vi "Update Tree.vi"(7 "Tree":refnum<vi>, 8 "error in (no error)":errorcluster, 11 "GenericGuiAI in":refnum<class "GenericGuiAI.lvclass">) -> (0 "error out":errorcluster, 3 "GenericGuiAI out":refnum<class "GenericGuiAI.lvclass">)   [LabVIEW 2020, in "VolatusDAQGenericGUI.lvlib" / "GenericGuiAI.lvclass"]
uses:
  GenericGuiAI.lvclass
  AI Tree Entry.ctl
  Channel Entry.ctl
  GenericGuiAI.lvclass/GenericGuiAI.ctl
  lv-vecto/Vecto/GroupAbstract/GroupAbstract.lvclass/GroupAbstract.ctl
  lv-vecto/Vecto/Channel/Channel.lvclass/Channel.ctl
  lv-vecto/Vecto/Group/Group.lvclass
  C:/dev/lv20CE/relink/lv-vecto/Vecto/GroupAbstract/GroupAbstract.lvclass
  lv-vecto/Vecto/GroupAbstract/Channel Info by Index.vi
  lv-vecto/Vecto/GroupAbstract/GroupAbstract.lvclass
  lv-vecto/Vecto/Group Config/Group Config.lvclass
  lv-vecto/Vecto/Channel/Channel.lvclass
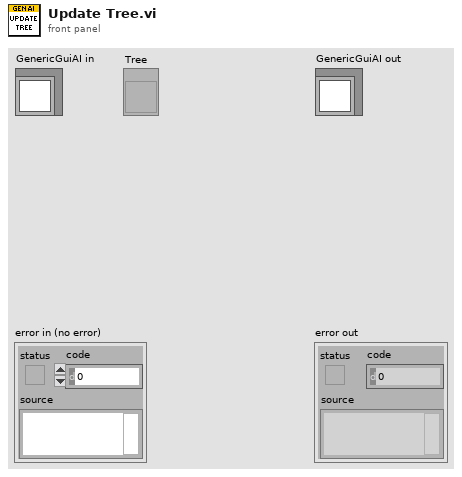
[diagram p1: front panel]
types:
  T1 = typedef "VolatusDAQGenericGUI.lvlib/GenericGuiAI.lvclass/AI Tree Entry.ctl" = cluster{"Hierarchy":string[], "Name":string, "Is Channel":bool, "Channel":T2}
  T2 = typedef "VolatusDAQGenericGUI.lvlib/GenericGuiAI.lvclass/Channel Entry.ctl" = cluster{"Resource":string, "Value":dbl, "Timestamp":dbl, "Raw":dbl}
  T3 = typedef "VectoConfig.lvlib/Group Info.ctl" = cluster{"System":string, "Cluster":string, "Node":string, "Task":string, "Name":string}
  T4 = typedef "VectoConfig.lvlib/Channel Info.ctl" = cluster{"Name":string, "Group":string, "Owning Node":string, "Owning Task":string, "Resource":string}
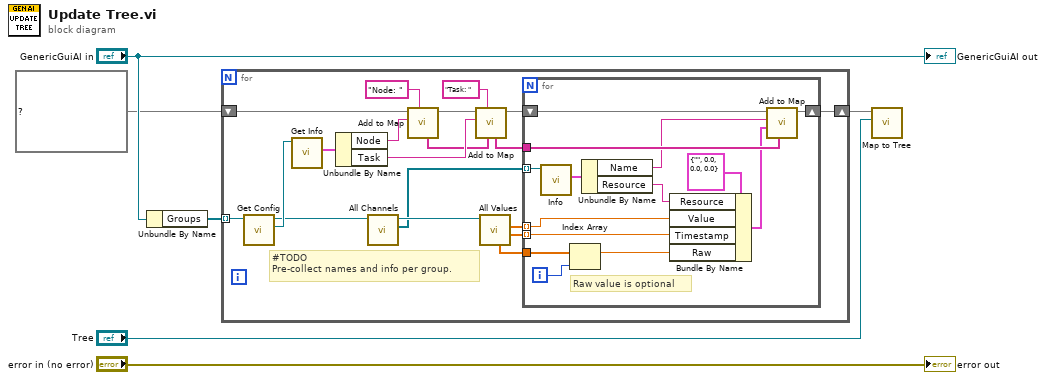
[diagram p0: block diagram]
diagram:
  n1 = Unbundle By Name("GenericGuiAI in") -> ("Groups"=w3:refnum<class "Group.lvclass">[])
  n2 = for {
    shift-right: [w10] -> w2
    shift-left: map{string[], T1} {} ("Map in") -> [w25]
    tunnel: w3 -> [w24] mode=indexing
    # "#TODO\nPre-collect names and info per group."
    n3 = call "Get Config.vi"("GroupAbstract in"=w24) -> ("Config"=w23:refnum<class "Group Config.lvclass">, "GroupAbstract out"=w9:refnum<class "Group.lvclass">)  [unwired: 8 in, 1 out]
    n4 = call "Get Info.vi"("Group Config in"=w23) -> ("Info"=w22:T3)  [unwired: 8 in, 2 out]
    n5 = Unbundle By Name(w22) -> ("Node"=w21:string, "Task"=w18:string)
    n6 = call "All Channels.vi"("Group in"=w9) -> ("All Channels"=w7:refnum<class "Channel.lvclass">[], "Group out"=w8:refnum<class "Group.lvclass">)  [unwired: 8 in, 1 out]
    n7 = call "Add to Map.vi"("Name Prefix (None)"="Node: ", "Name"=w21, "Map in"=w25) -> ("Map"=w19:map{string[], T1}, "Hierarchy"=w17:string[])  [unwired: 7 in]
    n8 = call "Add to Map.vi"("Parent (None)"=w17, "Name Prefix (None)"="Task: ", "Name"=w18, "Map in"=w19) -> ("Map"=w15:map{string[], T1}, "Hierarchy"=w14:string[])  [unwired: 6 in]
    n9 = call "All Values.vi"("Group in"=w8) -> ("Timestamp"=w12:dbl[], "Scaled"=w13:dbl[], "Raw"=w11:dbl[])  [unwired: 6 in, 2 out]
    n10 = for {
      shift-right: [w37] -> w10
      shift-left: w15 -> [w39]
      tunnel: w14 -> [w38]
      tunnel: w13 -> [w29] mode=indexing
      tunnel: w12 -> [w30] mode=indexing
      tunnel: w11 -> [w31]
      tunnel: w7 -> [w35] mode=indexing
      i -> [w26]
      # "Raw value is optional"
      n11 = call "Info.vi"("Channel in"=w35) -> ("Info"=w34:T4)  [unwired: 8 in, 2 out]
      n12 = Index Array(array=w31, index=w26) -> (element=w27:dbl)
      n13 = Unbundle By Name(w34) -> ("Name"=w33:string, "Resource"=w28:string)
      n14 = Bundle By Name(cluster=T2 {"Resource"="", "Value"=0.0, "Timestamp"=0.0, "Raw"=0.0} ("Channel (Not Channel)"), "Resource"=w28, "Value"=w29, "Timestamp"=w30, "Raw"=w27) -> (w32:T2)
      n15 = call "Add to Map.vi"("Parent (None)"=w38, "Channel (Not Channel)"=w32, "Name"=w33, "Map in"=w39) -> ("Map"=w37:map{string[], T1})  [unwired: 6 in, 1 out]
    }
  }
  n16 = call "Map to Tree.vi"("Tree"="Tree", "Map in"=w2) -> ()  [unwired: 10 in]
  "error out" <- "error in (no error)"
  "GenericGuiAI out" <- "GenericGuiAI in"
